vi "Experiment header-Get parameter names.vi"(8 "error in (no error)":errorcluster, 11 "Section Refs":T1[](array[typedef])) -> (0 "error out":errorcluster, 2 "All Parameter names":T2[](array[typedef]), 3 "Section Names":string[](array[string]))   [LabVIEW 2017]
uses:
  Typedefs/Header file parameter names.ctl
  Typedefs/Header file section refs.ctl
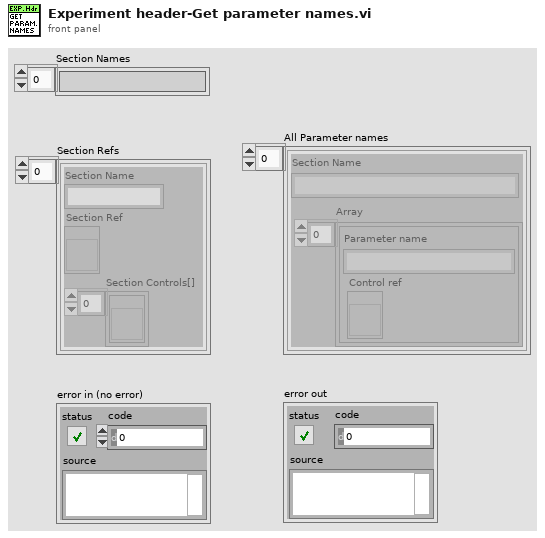
[diagram p1: front panel]
types:
  T1 = typedef "Header file section refs.ctl" = cluster{"Section Name":string, "Section Ref":refnum<vi>, "Section Controls[]":refnum<vi>[]}
  T2 = typedef "Header file parameter names.ctl" = cluster{"Section Name":string, "Array":cluster{"Parameter name":string, "Control ref":refnum<vi>}[]}
  T3 = cluster{"Parameter name":string, "Control ref":refnum<vi>}
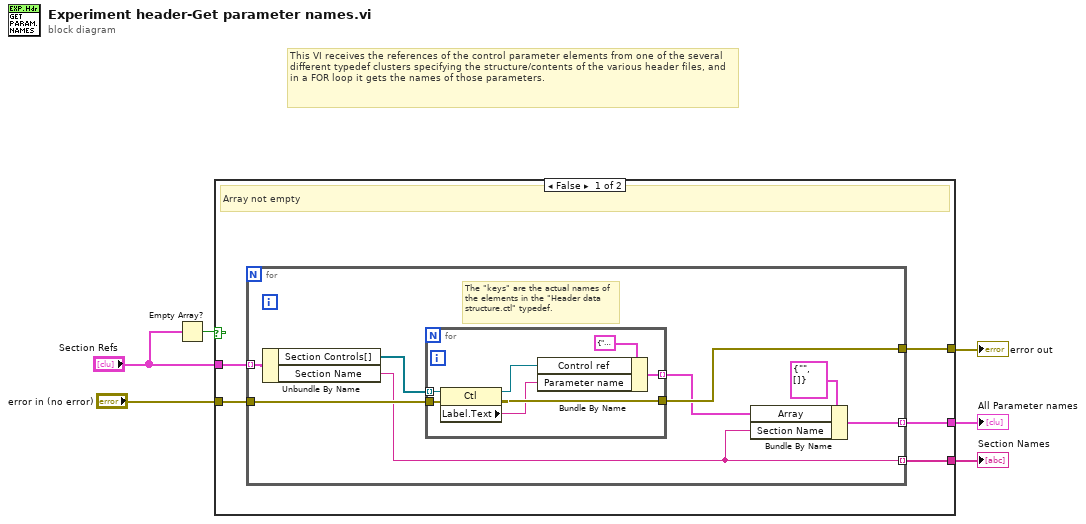
[diagram p0: block diagram]
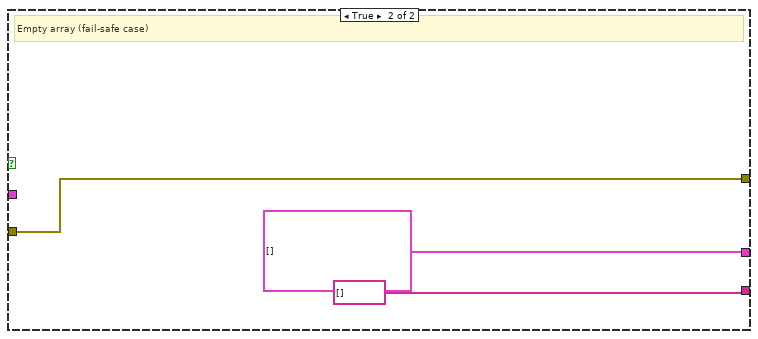
[diagram p2: hidden frame]
diagram:
  # "This VI receives the references of the control parameter elements from one of the several different typedef clusters specifying the structure/contents of the various header files, and in a FOR loop it gets the names of those parameters."
  n1 = Empty Array?(array="Section Refs") -> (empty?=w5:bool)
  n2 = case shown="False" w5 {
    tunnel: [w8 w29] -> w6
    tunnel: "error in (no error)" -> [w11 w29]
    tunnel: [w10 T2[] []] -> w4
    tunnel: "Section Refs" -> [w9 _]
    tunnel: [w7 string[] []] -> w1
    frame False {
      # "Array not empty"
      n3 = for {
        tunnel: w11 -> [w15]
        tunnel: [w18] -> w10 mode=indexing
        tunnel: w9 -> [w17] mode=indexing
        tunnel: [w14] -> w8
        tunnel: [w13] -> w7 mode=indexing
        # "The \"keys\" are the actual names of the elements in the \"Header data structure.ctl\" typedef."
        n4 = Unbundle By Name(w17) -> ("Section Controls[]"=w16:refnum<vi>[], "Section Name"=w13:string)
        n5 = for {
          tunnel: w16 -> [w26] mode=indexing
          tunnel: w15 -> [w25]
          tunnel: [w24] -> w14
          tunnel: [w20] -> w12 mode=indexing
          n6 = property on="Property Node" class="Ctl"(reference=w26, error in=w25) -> (reference out=w21:refnum<vi>, error out=w24:errorcluster, "Label.Text"=w22:string)
          n7 = Bundle By Name(cluster=T3 {"Parameter name"="", "Control ref"=refnum} ("Parameter name& ref"), "Control ref"=w21, "Parameter name"=w22) -> (w20:T3)
        }
        n8 = Bundle By Name(cluster=T2 {"Section Name"="", "Array"=[]} ("Parameter names"), "Array"=w12, "Section Name"=w13) -> (w18:T2)
      }
    }
    frame True {
      # "Empty array (fail-safe case)"
    }
  }
  "error out" <- w6
  "All Parameter names" <- w4
  "Section Names" <- w1
